vi "termLaser.vi"(8 "error in (no error)":errorcluster, 11 "connection ID":refnum<k5>) -> (0 "error out":errorcluster)   [LabVIEW 2018]
doc: "termLaser (Terminate Laser) close the connection between Keyence laser and labview via TCP."
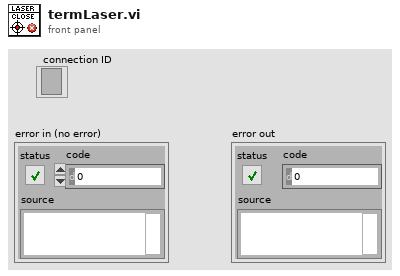
[diagram p1: front panel]
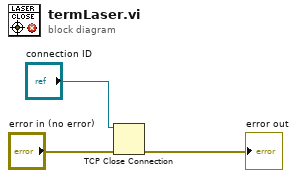
[diagram p0: block diagram]
diagram:
  n1 = TCP Close Connection(connection ID="connection ID", error in (no error)="error in (no error)") -> (error out=→"error out":errorcluster)  [unwired: 1 in, 1 out]
